vi "getIPR.vi"(6 "Address":i32=68, 8 "error in":errorcluster, 11 "connection ID":refnum<k5>) -> (0 "error out":errorcluster, 2 "Data":string, 3 "connection ID out":refnum<k5>, 5 "IPR_count":u32)   [LabVIEW 2012]
panel:
  in  "Data Read":bool=TRUE
  out "IPR_Data":string="0_2-0@0\r\n"
  out "Reg 65":string="0_2-0@0\r\n"
  out "Data READ":string="empty_read_buffer"
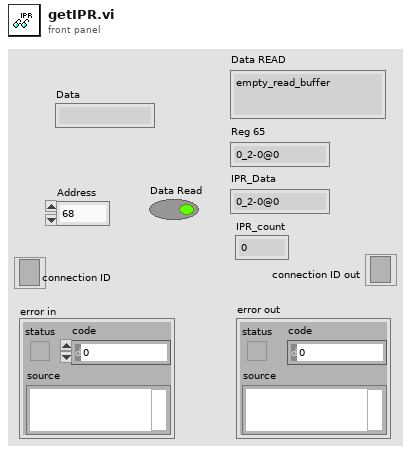
[diagram p1: front panel]
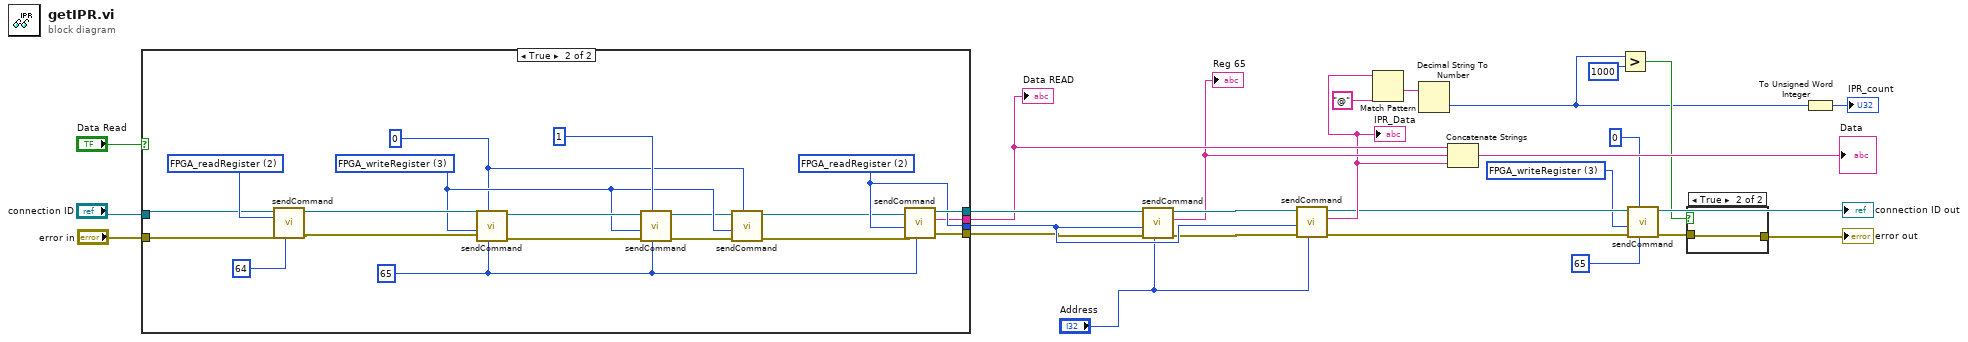
[diagram p0: block diagram]
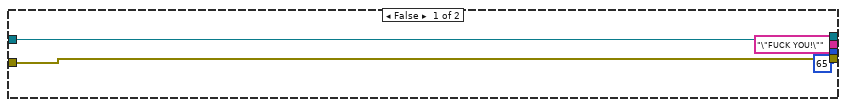
[diagram p3: hidden frame]
diagram:
  w10 = u16 3 items=["sendCommand"=9, "FPGA_writeRegister"=3, "FPGA_readRegister"=2, "uC_writeRegister"=1, "uC_readRegister"=0] ("Action")
  n1 = case shown="True" "Data Read" {
    tunnel: [w30 w51] -> w27
    tunnel: [u16 65 ("Action") w50] -> w25
    tunnel: "error in" -> [w31 w43]
    tunnel: "connection ID" -> [w30 w42]
    tunnel: ["\"FUCK YOU!\"" ("Data out") w47] -> w18
    tunnel: [w31 w45] -> w8
    frame False {
    }
    frame True {
      w44 = u16 2 items=["sendCommand"=9, "FPGA_writeRegister"=3, "FPGA_readRegister"=2, "uC_writeRegister"=1, "uC_readRegister"=0] ("Action")
      w46 = 65 ("Address")
      w37 = 0 ("Data")
      w38 = u16 3 items=["sendCommand"=9, "FPGA_writeRegister"=3, "FPGA_readRegister"=2, "uC_writeRegister"=1, "uC_readRegister"=0] ("Action")
      w50 = u16 2 items=["sendCommand"=9, "FPGA_writeRegister"=3, "FPGA_readRegister"=2, "uC_writeRegister"=1, "uC_readRegister"=0] ("Action")
      n2 = call "sendCommand.vi"("Address"=64, "error in"=w43, "Action"=w44, "connection ID"=w42) -> ("error out"=w33:errorcluster, "connection ID out"=w41:refnum<k5>)  [unwired: 3 in, 3 out]
      n3 = call "sendCommand.vi"("Address"=w46, "Data"=w37, "error in"=w33, "Action"=w38, "connection ID"=w41) -> ("error out"=w39:errorcluster, "connection ID out"=w48:refnum<k5>)  [unwired: 2 in, 3 out]
      n4 = call "sendCommand.vi"("Address"=w46, "Data"=1, "error in"=w39, "Action"=w38, "connection ID"=w48) -> ("error out"=w36:errorcluster, "connection ID out"=w35:refnum<k5>)  [unwired: 2 in, 3 out]
      n5 = call "sendCommand.vi"("Data"=w37, "error in"=w36, "Action"=w38, "connection ID"=w35) -> ("error out"=w32:errorcluster, "connection ID out"=w34:refnum<k5>)  [unwired: 3 in, 3 out]
      n6 = call "sendCommand.vi"("Address"=w46, "error in"=w32, "Action"=w50, "connection ID"=w34) -> ("error out"=w45:errorcluster, "Data out"=w47:string, "connection ID out"=w51:refnum<k5>)  [unwired: 3 in, 2 out]
    }
  }
  "Data READ" <- w18
  n7 = call "sendCommand.vi"("Address"="Address", "error in"=w8, "Action"=w25, "connection ID"=w27) -> ("error out"=w7:errorcluster, "Data out"=w17:string, "connection ID out"=w26:refnum<k5>)  [unwired: 3 in, 2 out]
  "Reg 65" <- w17
  n8 = call "sendCommand.vi"("Address"="Address", "error in"=w7, "Action"=w25, "connection ID"=w26) -> ("error out"=w6:errorcluster, "Data out"=w16:string, "connection ID out"=w13:refnum<k5>)  [unwired: 3 in, 2 out]
  "IPR_Data" <- w16
  n9 = Match Pattern(string=w16, regular expression="@" ("search string/char (-)")) -> (after substring=w22:string)  [unwired: 1 in, 3 out]
  n10 = Decimal String To Number(string=w22) -> (number=w4:i32)  [unwired: 2 in, 1 out]
  n11 = Concatenate Strings(w18, w17, w16) -> (→"Data":string)
  n12 = Greater?(x=w4, y=1000) -> (0:w5:bool)
  n13 = call "sendCommand.vi"("Address"=65, "Data"=0, "error in"=w6, "Action"=w10, "connection ID"=w13) -> ("error out"=w2:errorcluster, "connection ID out"=→"connection ID out":refnum<k5>)  [unwired: 2 in, 3 out]
  n14 = case shown="True" w5 {
    tunnel: [w52 w53] -> w1
    tunnel: w2 -> [w52 w53]
    frame False {
    }
    frame True {
    }
  }
  "error out" <- w1
  n15 = To Unsigned Word Integer(number=w4) -> (unsigned 16bit integer=→"IPR_count":u16)
